vi "subVI_ReadFMS_teleop.vi"(8 "error in (no error)":errorcluster) -> (0 "error out":errorcluster, 1 "Left":bool, 2 "AutoDriveCommand":string[](array[string]))   [LabVIEW 2017]
uses:
  <vilib>/Rock Robotics/Network Tables/NT Read String Array.vi
panel:
  out "substring":string
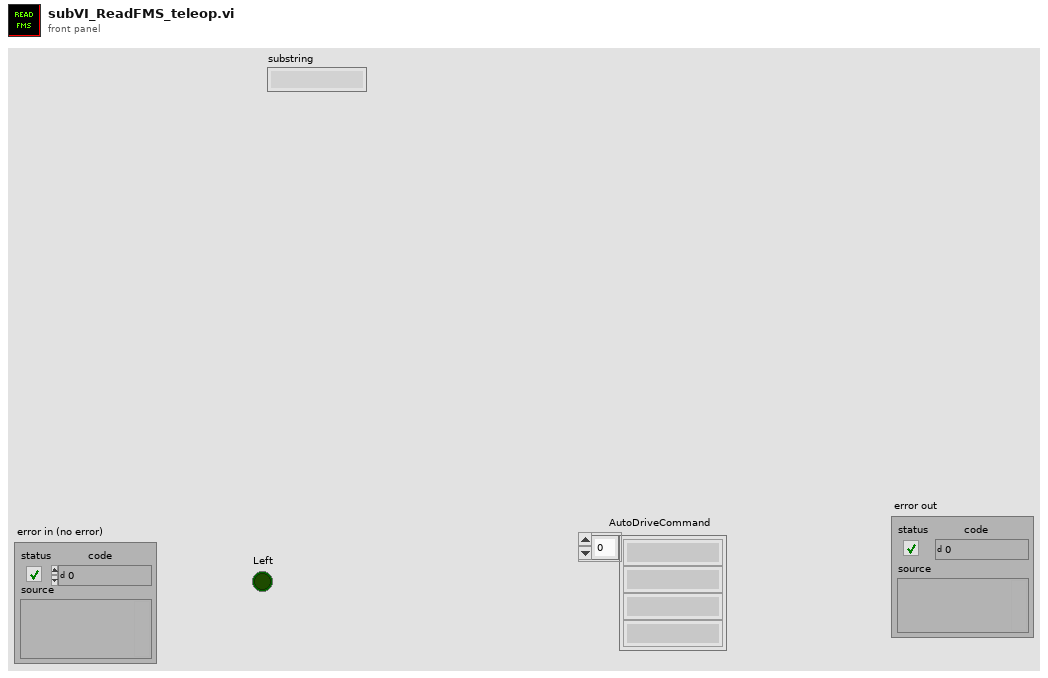
[diagram p1: front panel]
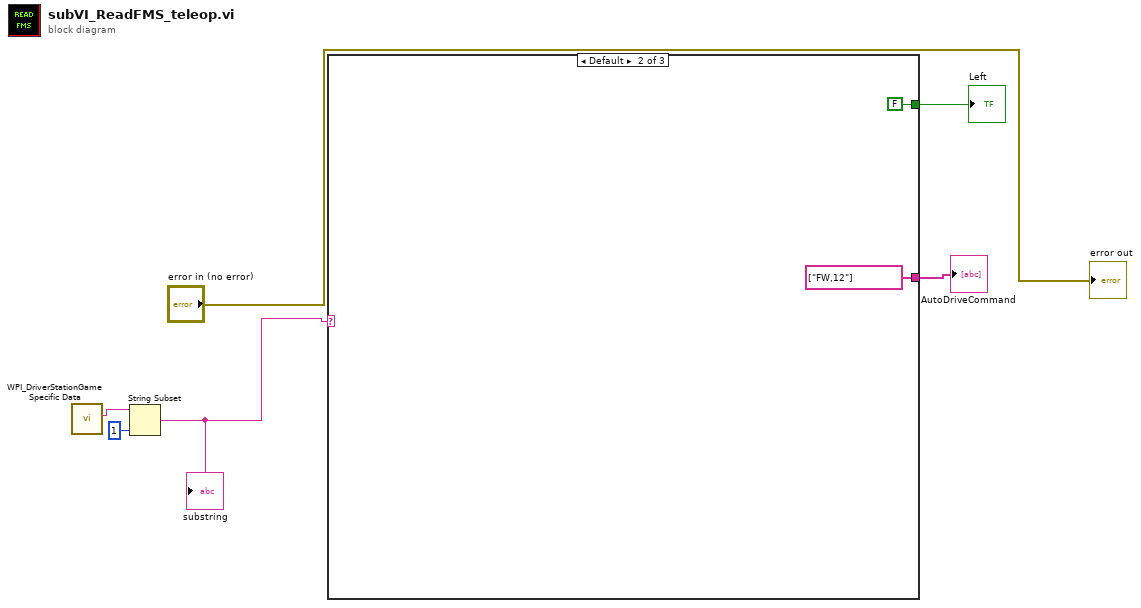
[diagram p0: block diagram]
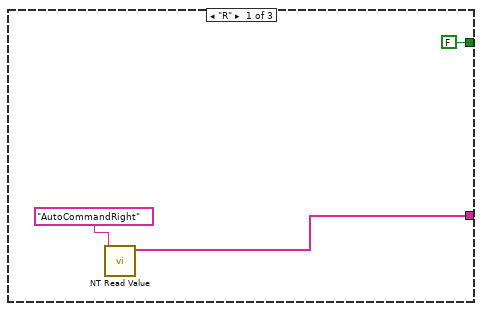
[diagram p2: hidden frame]
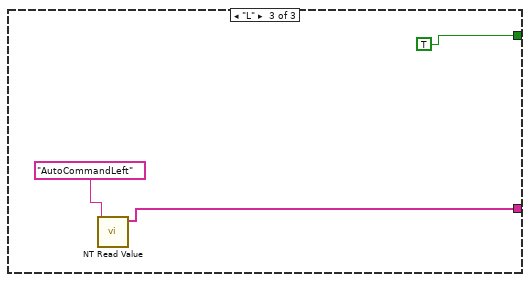
[diagram p3: hidden frame]
diagram:
  n1 = call <vilib>:"WPI_DriverStationGame Specific Data.vi"() -> ("Game Specific Data"=w6:string)  [unwired: 11 in]
  n2 = String Subset(string=w6, length (rest)=1 ("length (rest)")) -> (substring=w4:string)  [unwired: 1 in]
  "substring" <- w4
  n3 = case shown="Default" w4 {
    tunnel: [w8 string[] ["FW,12"] ("String Array") w13] -> w3
    tunnel: [FALSE ("Left") FALSE ("Left") TRUE ("Left")] -> w1
    frame "R" {
      n4 = call-poly <vilib>:"NT Read Value.vi"("Name"="AutoCommandRight") -> ("String Array"=w8:string[])  [unwired: 9 in, 1 out]
    }
    frame Default {
    }
    frame "L" {
      n5 = call-poly <vilib>:"NT Read Value.vi"("Name"="AutoCommandLeft") -> ("String Array"=w13:string[])  [unwired: 9 in, 1 out]
    }
  }
  "AutoDriveCommand" <- w3
  "Left" <- w1
  "error out" <- "error in (no error)"
